vi "SDCP BTR FGV.vi"(3 "error in (no error)":errorcluster, 4 "Command":enum16{"Read", "Write"}(ring), 5 "in":T1={"BTR_REQ"=FALSE, "BTR_ACK"=FALSE, "BTR_NPAR"=0, "BTR_NTR"=0, "BTR_PIDs"=[0, 0, 0, 0, 0, 0, 0, 0, 0]}) -> (0 "error out":errorcluster, 2 "out":T1)   [LabVIEW 2020]
uses:
  Typedefs/SDCP BTR Params.ctl
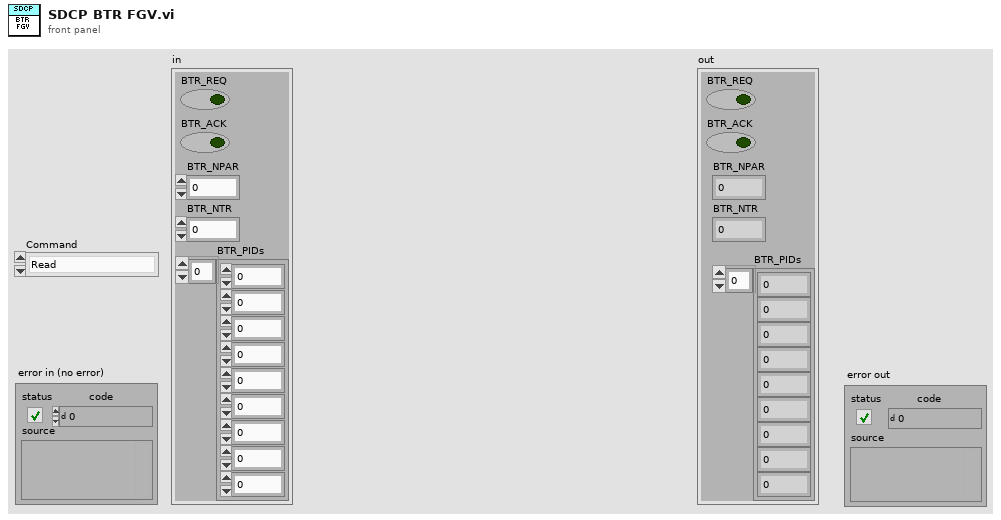
[diagram p1: front panel]
types:
  T1 = typedef "SDCP BTR Params.ctl" = cluster{"BTR_REQ":bool, "BTR_ACK":bool, "BTR_NPAR":i32, "BTR_NTR":i32, "BTR_PIDs":u8[]}
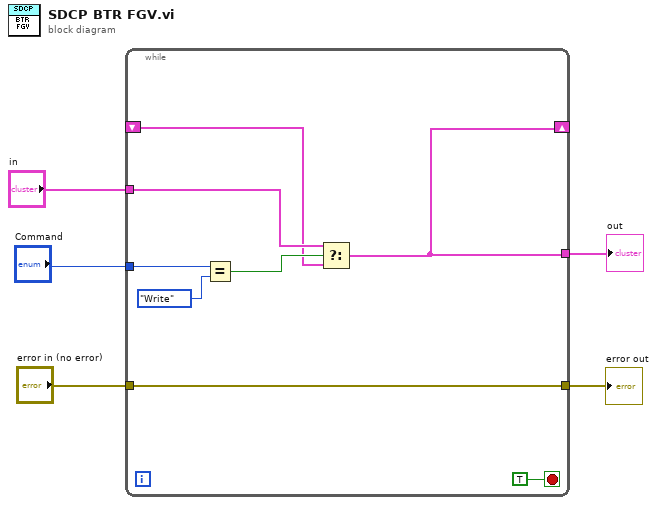
[diagram p0: block diagram]
diagram:
  n1 = while {
    tunnel: "error in (no error)" -> [w6]
    shift-right: [w7] -> _
    shift-left: _ -> [w8]
    tunnel: "Command" -> [w12]
    tunnel: "in" -> [w10]
    tunnel: [w7] -> w2
    tunnel: [w6] -> w1
    stop <- TRUE stop-if-true
    n2 = Equal?(x=w12, y=enum16{"Read", "Write"}."Write") -> (x = y?=w9:bool)
    n3 = Select(t=w10, s=w9, f=w8) -> (s? t:f=w7:T1)
  }
  "error out" <- w1
  "out" <- w2
